vi "LocalizeFromImageWithDebugOutput.vi"(0 "tracker":u64, 1 "xcor_iterations":i32=1, 2 "input image":T1, 3 "debug image":T1) -> (6 "tracker":u64, 7 "COM":cluster{"X":sgl, "Y":sgl}, 8 "debug image":T1(plugin-control), 9 "xcorpos":cluster{"X":sgl, " Y":sgl}, 10 "median":sgl=-1.0)   [LabVIEW 2011]
uses:
  <vilib>/vision/Image Controls.llb/IMAQ Image.ctl
  TrackerDLL.vi
panel:
  in  "XCor X":sgl
  in  "XCor Y":sgl
  in  "comX":sgl
  in  "comY":sgl
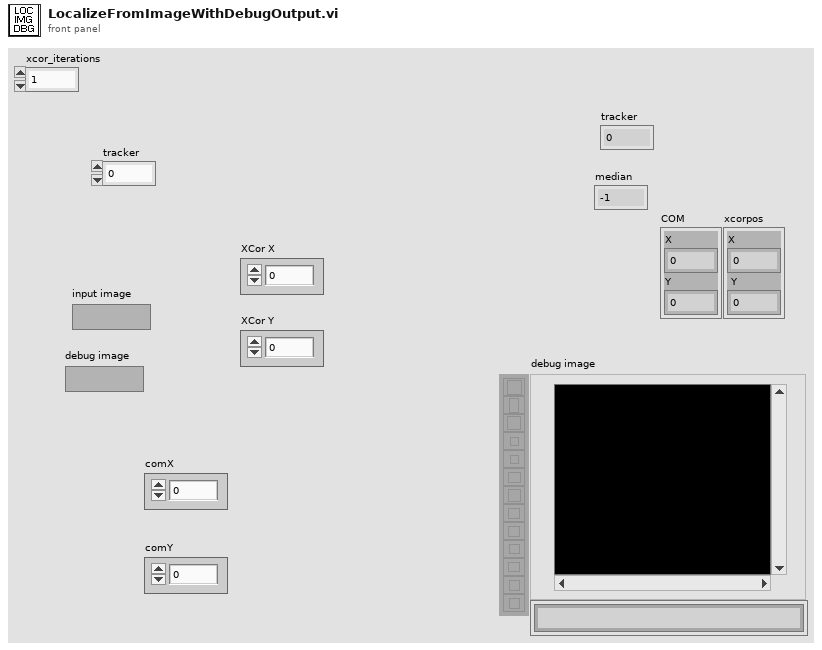
[diagram p1: front panel]
types:
  T1 = typedef "IMAQ Image.ctl" = refnum<image>
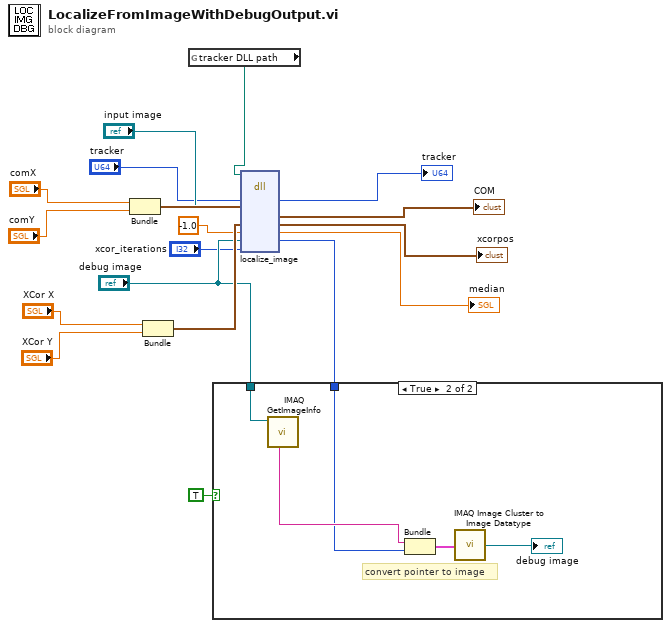
[diagram p0: block diagram]
diagram:
  n1 = Bundle("comX"="comX", "comY"="comY") -> (w16:cluster{"comX":sgl, "comY":sgl})  [unwired: 1 in]
  n2 = Bundle("XCor X"="XCor X", "XCor Y"="XCor Y") -> (w13:cluster{"XCor X":sgl, "XCor Y":sgl})  [unwired: 1 in]
  n3 = global read "TrackerDLL.vi" "tracker DLL path"() -> (w5:path)
  n4 = dll-call lib="D:/jcnossen1/cudaqi-tracker/Debug/cputrack.dll" fn="localize_image"(path in=w5, "tracker"="tracker", "image"="input image", "COM"=w16, "xcorpos"=w13, "median"=sgl -1.0, "debugImage"="debug image", "xcor_iterations"="xcor_iterations") -> ("tracker"=→"tracker":u64, "COM"=→"COM":cluster{"comX":sgl, "comY":sgl}, "xcorpos"=→"xcorpos":cluster{"XCor X":sgl, "XCor Y":sgl}, "median"=→"median":sgl, "debugImage"=w6:u64)  [unwired: 5 in, 2 out]
  n5 = case shown="True" TRUE {
    tunnel: "debug image" -> [_ w20]
    tunnel: w6 -> [_ w19]
    frame False {
    }
    frame True {
      # "convert pointer to image"
      n6 = call "IMAQ GetImageInfo"("Image"=w20) -> ("Image Name"=w21:string)  [unwired: 3 in, 7 out]
      n7 = Bundle("Image Name"=w21, "debugImage"=w19) -> (w22:cluster{"Image Name":string, "debugImage":u64})  [unwired: 1 in]
      n8 = call <vilib>:"IMAQ Image Cluster to Image Datatype.vi"("Image"=w22) -> ("Image (dup)"=→"debug image":T1)
    }
  }
